vi "BIO_new_socket.vi"(8 "error in (no error)":errorcluster, 9 "Close on free? (T)":bool=TRUE, 10 "fd":i32, 11 "SSL-Context in":refnum<class "SSL-Context.lvclass">) -> (0 "error out":errorcluster, 2 "Socket BIO out":refnum<class "BIO.lvclass">, 3 "SSL-Context out":refnum<class "SSL-Context.lvclass">)   [LabVIEW 2013, in "SSL_Lib.lvlib" / "SSL-Context.lvclass"]
uses:
  SSL-Context.lvclass
  BIO/BIO.lvclass
  SSL-Lib/SSL-Lib.lvclass/SSL-Lib.ctl
  BIO/BIO.lvclass/BIO.ctl
  SSL-Lib/Read Crypto Library Path.vi
  BIO/Write Handle.vi
  SSL-Lib/SSL-Lib.lvclass
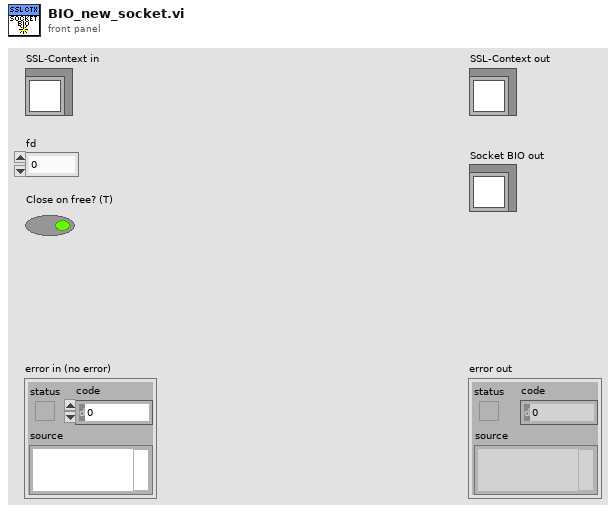
[diagram p1: front panel]
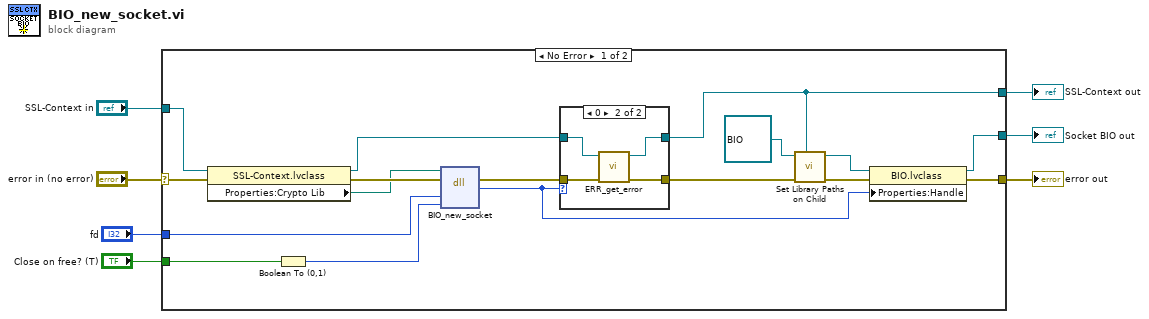
[diagram p0: block diagram]
diagram:
  n1 = case shown="No Error" "error in (no error)" {
    selector: "error in (no error)" -> [w24 w32]
    tunnel: [w17 w32] -> w6
    tunnel: [w13 w31] -> w4
    tunnel: "SSL-Context in" -> [w22 w31]
    tunnel: [w16 _] -> w3
    tunnel: "Close on free? (T)" -> [w10 _]
    tunnel: "fd" -> [w8 _]
    frame No Error {
      n2 = property class="SSL-Context.lvclass"(reference=w22, error in=w24) -> (reference out=w14:refnum<class "SSL-Context.lvclass">, error out=w23:errorcluster, "Properties:Crypto Lib"=w21:path)
      n3 = Boolean To (0,1)(Boolean=w10) -> (0, 1=w9:i16)
      n4 = dll-call lib="C:/Program Files (x86)/National Instruments/Shared/nissl/NIlibeay32.dll" fn="BIO_new_socket"(path in=w21, error in=w23, "fd"=w8, "c"=w9) -> (error out=w15:errorcluster, "return type"=w11:u64)  [unwired: 3 in, 1 out]
      n5 = case shown="0" w11 {
        tunnel: w15 -> [w26 w30]
        tunnel: w14 -> [w25 w29]
        tunnel: [w25 w28] -> w13
        tunnel: [w26 w27] -> w12
        frame Default {
        }
        frame 0 {
          n6 = call "ERR_get_error.vi"("error in (no error)"=w30, "SSL-Lib in"=w29) -> ("error out"=w27:errorcluster, "SSL-Lib out"=w28:refnum<class "SSL-Context.lvclass">)  [unwired: 8 in]
        }
      }
      n7 = call-dynamic "Set Library Paths on Child.vi"(7:"SSL-Lib in"=w13, "error in (no error)"=w12, 11:"SSL-Lib in"=refnum<class "BIO.lvclass"> refnum ("SSL_Lib.lvlib:BIO.lvclass")) -> ("error out"=w19:errorcluster, "SSL-Lib out"=w18:refnum<class "BIO.lvclass">)  [unwired: 7 in]
      n8 = property class="BIO.lvclass"(reference=w18, error in=w19, "Properties:Handle"=w11) -> (reference out=w16:refnum<class "BIO.lvclass">, error out=w17:errorcluster)
    }
    frame Error {
    }
  }
  "error out" <- w6
  "SSL-Context out" <- w4
  "Socket BIO out" <- w3
